vi "ddsIterConvert.vi"(7 "Pre 3.0 AOM driver version?":bool, 10 "Register":dbl=11.0 min=0.0 max=16.0 step=1.0 format="%#.1f", 11 "Max Iterations":dbl=2.0 min=0.0 max=1023.0 step=1.0 format="%#.1f") -> (3 "Characters for FPGA":string="L;002\r\n")   [LabVIEW 2013, in "DDS9954_v2013.lvlib"]
uses:
  DDS9954_v2013.lvlib
  dataToAscii_16bit.vi
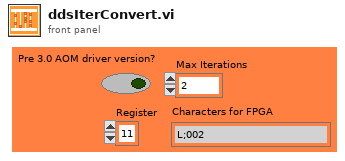
[diagram p1: front panel]
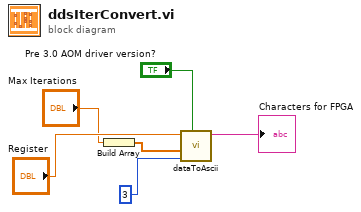
[diagram p0: block diagram]
diagram:
  n1 = Build Array("Max Iterations") -> (w3:dbl[])
  n2 = call-poly "dataToAscii.vi"("Pre 3.0 AOM driver version?"="Pre 3.0 AOM driver version?", "HEX min width (pre 3.0)"=u8 3, "Input Data"=w3, "Register"="Register") -> ("Characters to FPGA"=→"Characters for FPGA":string)  [unwired: 7 in]
